vi "List Files.vi"(0 "path":path, 1 "pattern (e.g. *.txt)":string, 11 "error in":errorcluster) -> (4 "path out":path, 6 "filenames":string[](array[string]), 8 "filesizes (bytes)":i64[](array[numeric]), 10 "last modificadtion data":timestamp[](array[timestamp]), 14 "# of files":i32, 15 "error out":errorcluster)   [LabVIEW 2019]
doc: "List Files in a folder."
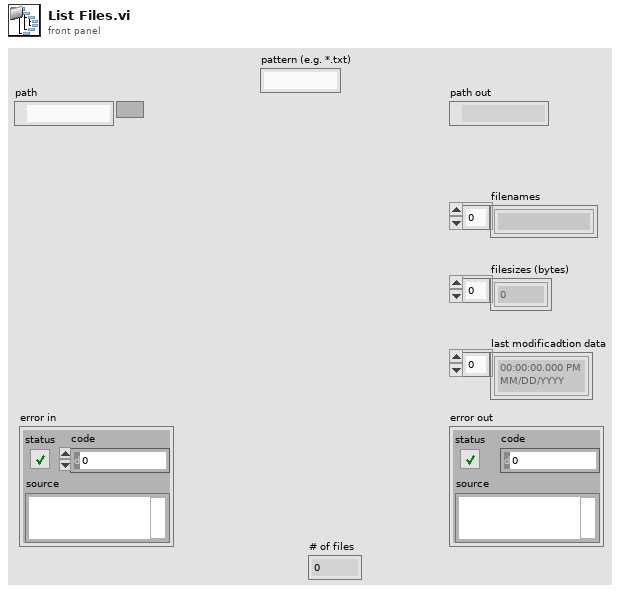
[diagram p1: front panel]
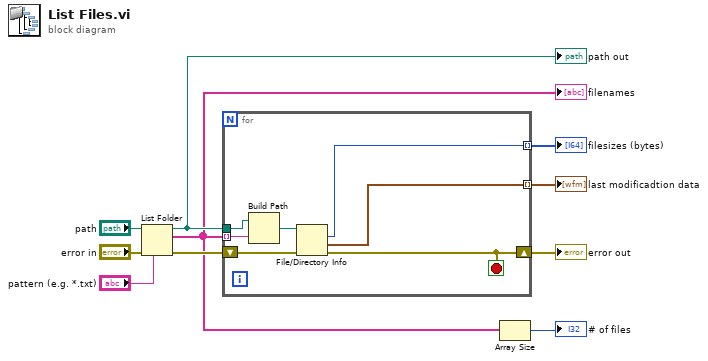
[diagram p0: block diagram]
diagram:
  n1 = List Folder(path="path", pattern="pattern (e.g. *.txt)", error in="error in") -> (path out=w5:path, filenames=w3:string[], error out=w7:errorcluster)  [unwired: 1 in, 1 out]
  "filenames" <- w3
  "path out" <- w5
  n2 = for {
    shift-right: [w12] -> w6
    shift-left: w7 -> [w13]
    tunnel: [w14] -> w4 mode=indexing
    tunnel: w3 -> [w17] mode=indexing
    tunnel: w5 -> [w16]
    tunnel: [w11] -> w1 mode=indexing
    stop <- w12 stop-if-true
    n3 = Build Path(base path=w16, name or relative path=w17) -> (appended path=w15:path)
    n4 = File/Directory Info(path=w15, error in=w13) -> (size=w14:i64, last mod=w11:timestamp, error out=w12:errorcluster)  [unwired: 4 out]
  }
  "error out" <- w6
  "filesizes (bytes)" <- w4
  "last modificadtion data" <- w1
  n5 = Array Size(array=w3) -> (size(s)=→"# of files":i32)
